vi "Test Display Panel V3 Multiple.vi"() -> ()   [LabVIEW 2014, in "Display Panel.lvlib" / "Display Panel V3.lvclass"]
uses:
  Display Panel V3.lvclass
  <vilib>/ActorFramework/Message Enqueuer/Message Enqueuer.lvclass
  <vilib>/ActorFramework/Message Queue/Message Queue.lvclass/Message Queue.ctl
  Display Panel V3 Messages/Write Card Number From Control Msg/Write Card Number From Control Msg.lvclass/Write Card Number From Control Msg.ctl
  <vilib>/ActorFramework/Message Enqueuer/Message Enqueuer.lvclass/Message Enqueuer.ctl
  Display Panel V3 Messages/Insert into SubPanel Msg/Insert into SubPanel Msg.lvclass/Insert into SubPanel Msg.ctl
  <vilib>/ActorFramework/Message Enqueuer/Enqueue.vi
  <vilib>/ActorFramework/Message Priority Queue/Priority Enqueue.vi
  Display Panel V3 Messages/Write Card Number From Control Msg/Write Card Number From Control Msg.lvclass
  Display Panel V3 Messages/Insert into SubPanel Msg/Insert into SubPanel Msg.lvclass
  <vilib>/ActorFramework/Stop Msg/Stop Msg.lvclass
  <vilib>/ActorFramework/Message Queue/Message Queue.lvclass
  <vilib>/ActorFramework/Actor/Actor.lvclass
panel:
  out "size(s)":i32
  out "error out 2":errorcluster
  out "error out":errorcluster
  in  "Stop Button":bool
  in  "Menu Ring":u16(ring) items=["0", "1", "2"]
  out "Actor Enqueuers":refnum<class "Message Enqueuer.lvclass">[](array[class])
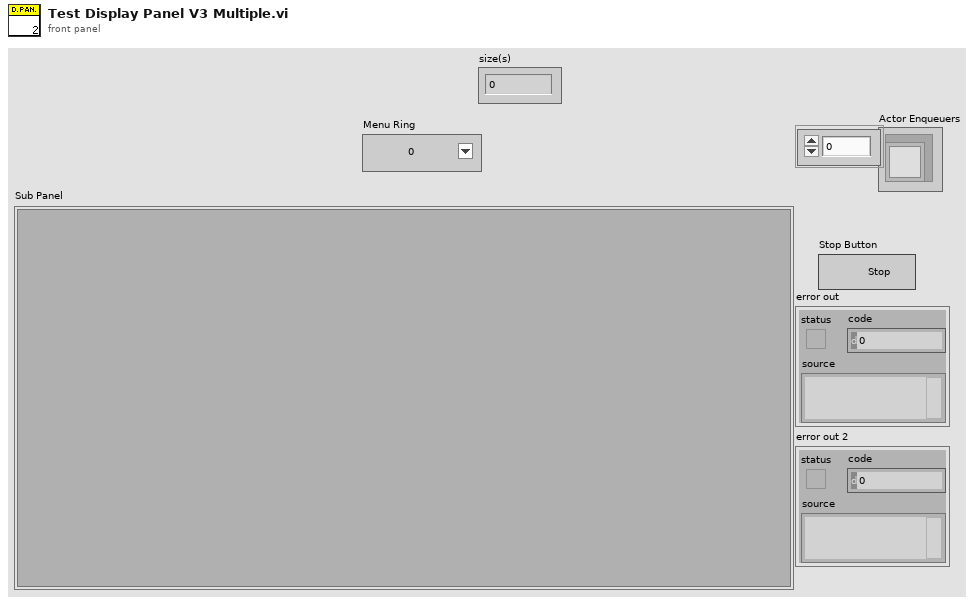
[diagram p1: front panel]
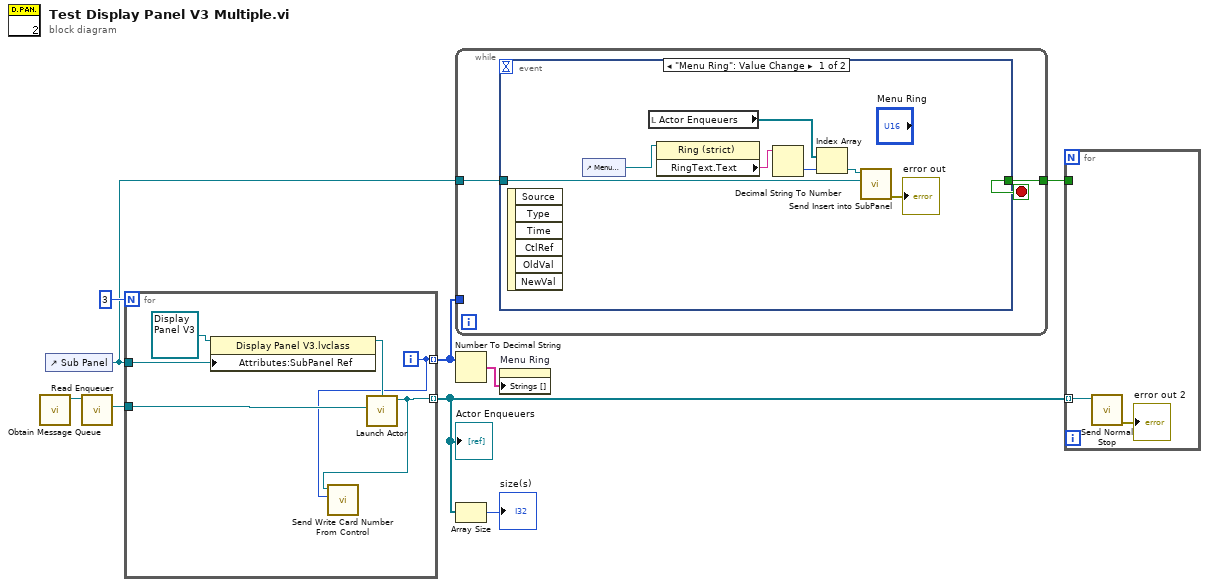
[diagram p0: block diagram]
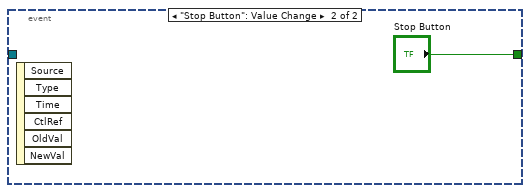
[diagram p2: hidden frame]
diagram:
  n1 = call <vilib>:"Obtain Message Queue.vi"() -> ("Message Queue"=w9:refnum<class "Message Queue.lvclass">)  [unwired: 10 in, 1 out]
  n2 = control-ref of="Sub Panel"() -> (w5:refnum<vi>)
  n3 = call <vilib>:"Read Enqueuer.vi"("Message Queue"=w9) -> ("Message Enqueuer"=w8:refnum<class "Message Enqueuer.lvclass">)  [unwired: 10 in]
  n4 = for {
    N: 3 -> [_]
    tunnel: w5 -> [w15]
    tunnel: w8 -> [w14]
    tunnel: [w11] -> w2 mode=indexing
    tunnel: [w10] -> w3 mode=indexing
    i -> [w10]
    n5 = property class="Display Panel V3.lvclass"(reference=refnum<class "Display Panel V3.lvclass"> refnum ("Display Panel.lvlib:Display Panel V3.lvclass"), "Attributes:SubPanel Ref"=w15) -> (reference out=w13:refnum<class "Display Panel V3.lvclass">)  [unwired: 1 in, 1 out]
    n6 = call <vilib>:"Launch Actor.vi"("Actor-to-Caller Enqueuer"=w14, "Actor"=w13) -> ("Caller-To-Actor Enqueuer"=w11:refnum<class "Message Enqueuer.lvclass">)  [unwired: 8 in, 1 out]
    n7 = call "Send Write Card Number From Control.vi"("Card Number"=w10, "Message Enqueuer"=w11) -> ()  [unwired: 8 in, 2 out]
  }
  "Actor Enqueuers" <- w2
  n8 = while {
    tunnel: w5 -> [w17]
    tunnel: [w16] -> w4
    tunnel: w3 -> [_]
    stop <- w16 stop-if-true
    n9 = event shown="[0] \"Menu Ring\": Value Change" {
      selector: _ -> [_ _]
      dyn-events: _ -> [_ _]
      timeout: _ -> [_ _]
      tunnel: w17 -> [w19 _]
      tunnel: [_ "Stop Button"] -> w16
      event "Menu Ring": Value Change {
        n10 = event-data() -> ()  [unwired: 1 in, 6 out]
        n11 = control-ref of="Menu Ring"() -> (w24:refnum<vi>)
        n12 = local read "Actor Enqueuers"() -> (w22:refnum<class "Message Enqueuer.lvclass">[])
        n13 = property class="Ring (strict)"(reference=w24) -> ("RingText.Text"=w23:string)  [unwired: 1 in, 2 out]
        n14 = Decimal String To Number(string=w23) -> (number=w21:i32)  [unwired: 2 in, 1 out]
        n15 = Index Array(array=w22, index=w21) -> (element=w20:refnum<class "Message Enqueuer.lvclass">)
        n16 = call "Send Insert into SubPanel.vi"("SubPanel Ref"=w19, "Message Enqueuer"=w20) -> ("error out"=→"error out":errorcluster)  [unwired: 8 in, 1 out]
      }
      event "Stop Button": Value Change {
        n17 = event-data() -> ()  [unwired: 1 in, 6 out]
      }
    }
  }
  n18 = Number To Decimal String(number=w3) -> (decimal integer string=w6:string[])  [unwired: 1 in]
  n19 = Array Size(array=w2) -> (size(s)=→"size(s)":i32)
  n20 = property on="Menu Ring" class="Ring (strict)"("Strings []"=w6) -> ()  [unwired: 2 in, 2 out]
  n21 = for {
    tunnel: w2 -> [w27] mode=indexing
    tunnel: w4 -> [_]
    n22 = call <vilib>:"Send Normal Stop.vi"("Message Enqueuer"=w27) -> ("error out"=→"error out 2":errorcluster)  [unwired: 10 in]
  }
